vi "Initialize Inline Buffer.vi"(8 "error in (no error)":errorcluster, 9 "size":u64 format="%d bytes", 10 "address":u64 format="%016x", 11 "Framework in":refnum<class "Framework.lvclass">) -> (0 "error out":errorcluster, 3 "Framework out":refnum<class "Framework.lvclass">)   [LabVIEW 2020, in "DSF Core.lvlib" / "Framework.lvclass"]
uses:
  Framework.lvclass
  <vilib>/NI/Memory Manager/Classes/Pointer/Pointer.lvclass
  Buffer/Buffer.lvclass
  C:/Program Files (x86)/National Instruments/LabVIEW 2020/vi.lib/NI/Memory Manager/Classes/Pointer/Pointer.lvclass
  C:/Users/nitest/Desktop/Git/niveristand-data-sharing-framework-custom-device/Source/Core/Classes/Buffer/Buffer.lvclass
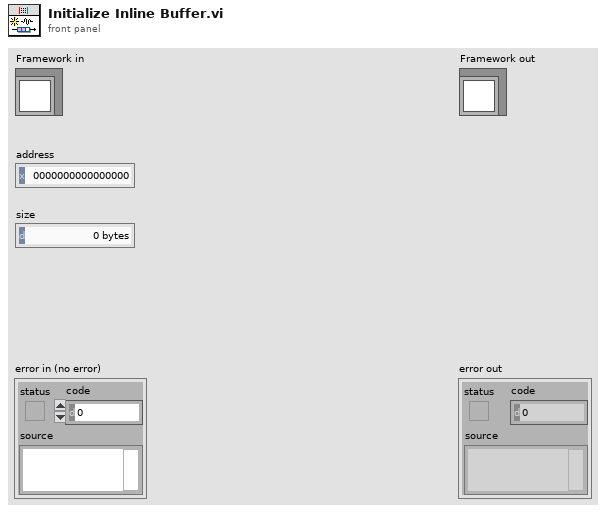
[diagram p1: front panel]
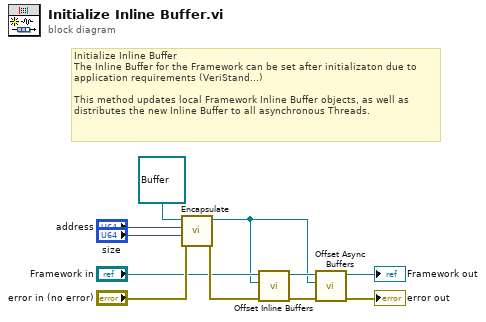
[diagram p0: block diagram]
diagram:
  # "Initialize Inline Buffer\nThe Inline Buffer for the Framework can be set after initializaton due to application requirements (VeriStand...)\n\nThis method updates local Framework Inline Buffer objects, as well as distributes the new Inline Buffer to all asynchronous Threads."
  n1 = call <vilib>:"Encapsulate.vi"("error in (no error)"="error in (no error)", "size"="size", "address"="address", "Pointer type"=refnum<class "Buffer.lvclass"> refnum ("Inline Buffer")) -> ("error out"=w4:errorcluster, "Pointer"=w1:refnum<class "Buffer.lvclass">)  [unwired: 6 in]
  n2 = call "Offset Inline Buffers.vi"("error in (no error)"=w4, "base Inline Buffer"=w1, "Framework in"="Framework in") -> ("error out"=w8:errorcluster, "Framework out"=w9:refnum<class "Framework.lvclass">)  [unwired: 7 in]
  n3 = call "Offset Async Buffers.vi"("error in (no error)"=w8, "base Inline Buffer"=w1, "Framework in"=w9) -> ("error out"=→"error out":errorcluster, "Framework out"=→"Framework out":refnum<class "Framework.lvclass">)  [unwired: 7 in]
